vi "ExtractStep.vi"(8 "error in (no error)":errorcluster, 11 "Internal Data":T2) -> (0 "error out":errorcluster, 3 "Zone Indicators Default":T1)   [LabVIEW 2019]
uses:
  Controls/InternalData.ctl
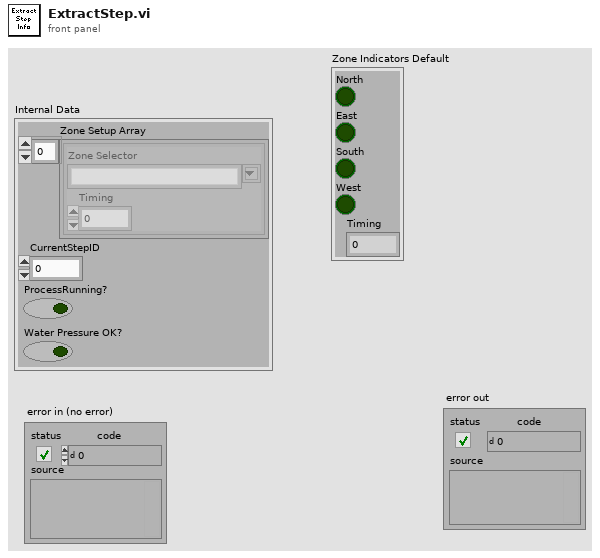
[diagram p1: front panel]
types:
  T1 = cluster{"North":bool, "East":bool, "South":bool, "West":bool, "Timing":u32}
  T2 = typedef "InternalData.ctl" = cluster{"Zone Setup Array":cluster{"Zone Selector":string, "Timing":dbl}[], "CurrentStepID":u32, "ProcessRunning?":bool, "Water Pressure OK?":bool}
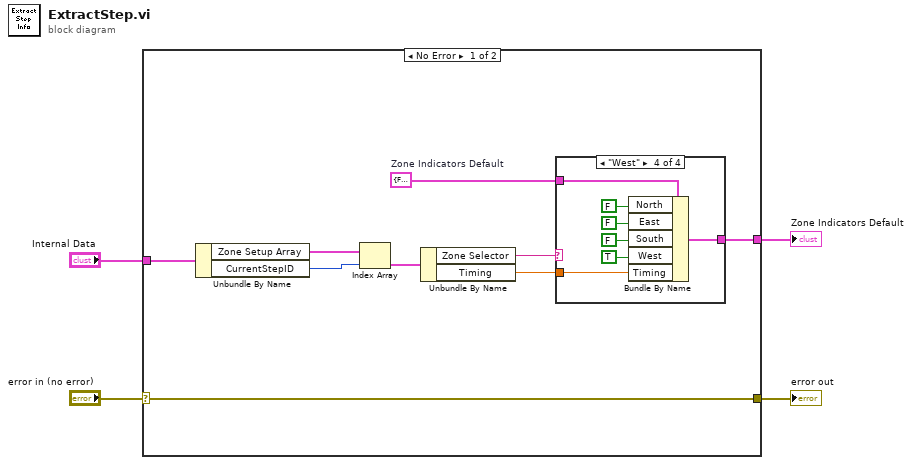
[diagram p0: block diagram]
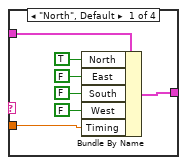
[diagram p2: hidden frame]
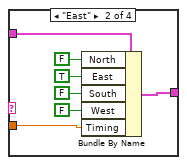
[diagram p3: hidden frame]
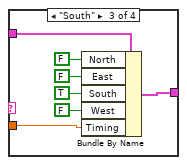
[diagram p4: hidden frame]
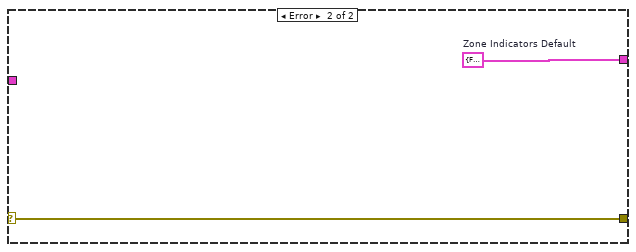
[diagram p5: hidden frame]
diagram:
  n1 = case shown="No Error" "error in (no error)" {
    selector: "error in (no error)" -> [w5 w43]
    tunnel: "Internal Data" -> [w13 _]
    tunnel: [w7 w42] -> w3
    tunnel: [w5 w43] -> w1
    frame No Error {
      w6 = T1 {"North"=FALSE, "East"=FALSE, "South"=FALSE, "West"=FALSE, "Timing"=0}  # Zone Indicators Default
      n2 = Unbundle By Name(w13) -> ("Zone Setup Array"=w12:cluster{"Zone Selector":string, "Timing":dbl}[], "CurrentStepID"=w11:u32)
      n3 = Index Array(array=w12, index=w11) -> (element=w10:cluster{"Zone Selector":string, "Timing":dbl})
      n4 = Unbundle By Name(w10) -> ("Zone Selector"=w9:string, "Timing"=w8:dbl)
      n5 = case shown="\"West\"" w9 {
        tunnel: w8 -> [w15 w22 w29 w36]
        tunnel: [w14 w21 w28 w35] -> w7
        tunnel: w6 -> [w20 w27 w34 w41]
        frame "North", Default {
          n6 = Bundle By Name(cluster=w20, "North"=TRUE, "East"=FALSE, "South"=FALSE, "West"=FALSE, "Timing"=w15) -> (w14:T1)
        }
        frame "East" {
          n7 = Bundle By Name(cluster=w27, "North"=FALSE, "East"=TRUE, "South"=FALSE, "West"=FALSE, "Timing"=w22) -> (w21:T1)
        }
        frame "South" {
          n8 = Bundle By Name(cluster=w34, "North"=FALSE, "East"=FALSE, "South"=TRUE, "West"=FALSE, "Timing"=w29) -> (w28:T1)
        }
        frame "West" {
          n9 = Bundle By Name(cluster=w41, "North"=FALSE, "East"=FALSE, "South"=FALSE, "West"=TRUE, "Timing"=w36) -> (w35:T1)
        }
      }
    }
    frame Error {
      w42 = T1 {"North"=FALSE, "East"=FALSE, "South"=FALSE, "West"=FALSE, "Timing"=0}  # Zone Indicators Default
    }
  }
  "Zone Indicators Default" <- w3
  "error out" <- w1
